vi "Read NumberOfTactics.vi"(8 "error in (no error)":errorcluster, 11 "ABCSecondKicker in":refnum<class "ABCSecondKicker.lvclass">) -> (0 "error out":errorcluster, 2 "NumberOfTactics":dbl=3.0, 3 "ABCSecondKicker out":refnum<class "ABCSecondKicker.lvclass">)   [LabVIEW 2021, in "ABCSecondKicker.lvclass"]
uses:
  ABCSecondKicker.lvclass
  ABCSecondKicker.lvclass/ABCSecondKicker.ctl
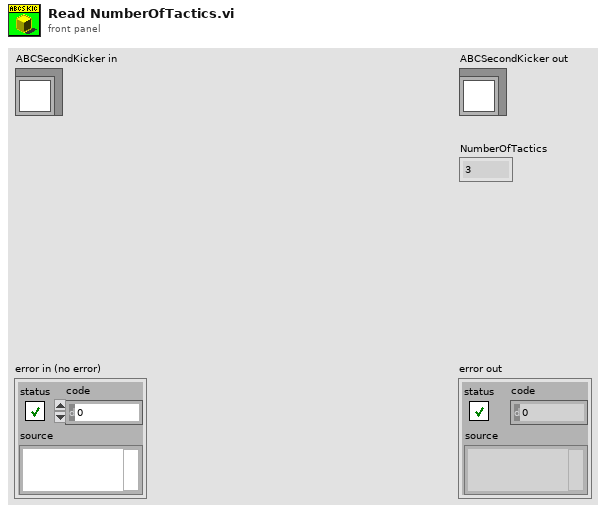
[diagram p1: front panel]
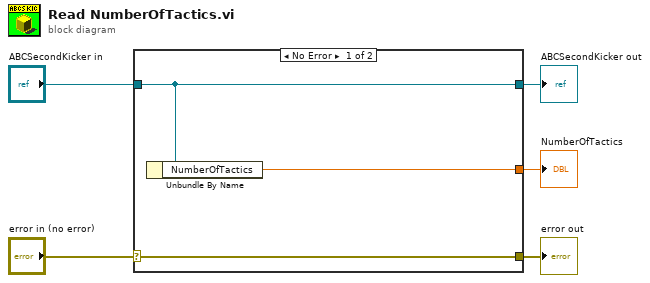
[diagram p0: block diagram]
diagram:
  n1 = case shown="No Error" "error in (no error)" {
    selector: "error in (no error)" -> [w8 w9]
    tunnel: [w8 w9] -> w4
    tunnel: [w7 w10] -> w2
    tunnel: "ABCSecondKicker in" -> [w7 w10]
    tunnel: [w6 _] -> w1
    frame No Error {
      n2 = Unbundle By Name(w7) -> ("NumberOfTactics"=w6:dbl)
    }
    frame Error {
    }
  }
  "error out" <- w4
  "ABCSecondKicker out" <- w2
  "NumberOfTactics" <- w1
